vi "VP_String.vi"(1 "Odour bottles":T1(array[cluster])) -> (0 "Odour bottles 2":T1(array[cluster]))   [LabVIEW 2016]
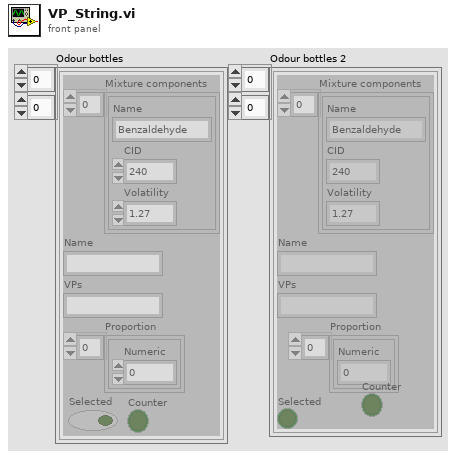
[diagram p1: front panel]
types:
  T1 = cluster{"Mixture components":cluster{"Name":string, "CID":i32, "Volatility":dbl}[], "Name":string, "VPs":string, "Proportion":cluster{"Numeric":dbl}[], "Selected":bool, "Counter":bool}[][]
  T2 = cluster{"Name":string, "CID":i32, "Volatility":dbl}[]
  T3 = cluster{"Mixture components":cluster{"Name":string, "CID":i32, "Volatility":dbl}[], "Name":string, "VPs":string, "Proportion":cluster{"Numeric":dbl}[], "Selected":bool, "Counter":bool}
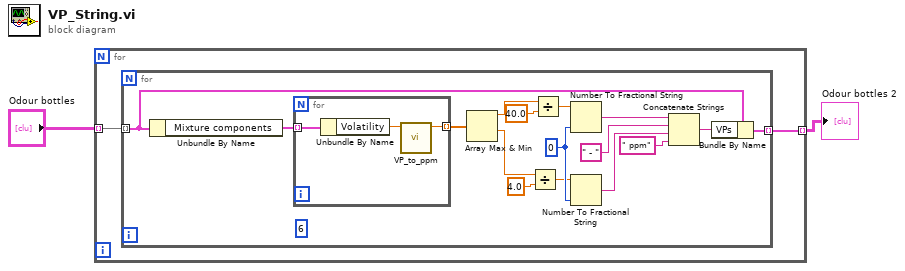
[diagram p0: block diagram]
diagram:
  n1 = for {
    tunnel: "Odour bottles" -> [w4] mode=indexing
    tunnel: [w3] -> w1 mode=indexing
    n2 = for {
      tunnel: w4 -> [w20] mode=indexing
      tunnel: [w17] -> w3 mode=indexing
      (unwired) i16 6 ("precision (6)")
      w13 = i16 0 ("precision (6)")
      n3 = Unbundle By Name(w20) -> ("Mixture components"=w19:T2)
      n4 = for {
        tunnel: w19 -> [w23] mode=indexing
        tunnel: [w21] -> w12 mode=indexing
        n5 = Unbundle By Name(w23) -> ("Volatility"=w22:dbl)
        n6 = call "VP_to_ppm.vi"("VP (Hgmm)"=w22) -> ("Saturated concentration (ppm)"=w21:dbl)  [unwired: 10 in]
      }
      n7 = Array Max & Min(array=w12) -> (max value=w11:dbl, min value=w8:dbl)  [unwired: 2 out]
      n8 = Divide(x=w8, y=4.0) -> (x/y=w6:dbl)
      n9 = Divide(x=w11, y=40.0) -> (x/y=w7:dbl)
      n10 = Number To Fractional String(number=w7, precision (6)=w13) -> (F-format string=w15:string)  [unwired: 2 in]
      n11 = Number To Fractional String(number=w6, precision (6)=w13) -> (F-format string=w14:string)  [unwired: 2 in]
      n12 = Concatenate Strings(w15, " - " ("string"), w14, " ppm" ("string")) -> (w18:string)
      n13 = Bundle By Name(cluster=w20, "VPs"=w18) -> (w17:T3)
    }
  }
  "Odour bottles 2" <- w1
